vi "start_sweep.vi"(8 "error in (no error)":errorcluster, 11 "ScanModeDL090923Scaffold in":refnum<class "ImagingModeDL090923Scaffold.lvclass">) -> (0 "error out":errorcluster, 3 "ScanModeDL090923Scaffold out":refnum<class "ImagingModeDL090923Scaffold.lvclass">)   [LabVIEW 2010, in "ImagingModeDL090923Scaffold.lvclass"]
uses:
  ImagingModeDL090923Scaffold.lvclass
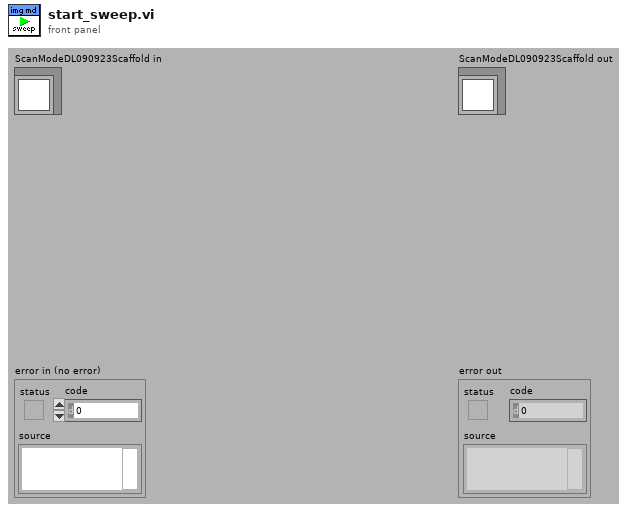
[diagram p1: front panel]
types:
  T1 = typedef "GenericToplevelComponent.lvclass/common_trigger_enum.ctl" = enum16{"NULL", "initialise", "terminate", "fetch command", "fetch data", "attach observer", "register as observer", "detach observer", "acknowledge", "start", "stop", "sweep started", "sweep finished", "experiment started", "experiment stopped"}
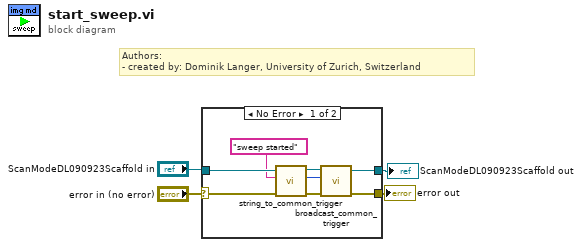
[diagram p0: block diagram]
diagram:
  # "Authors: \n- created by: Dominik Langer, University of Zurich, Switzerland"
  n1 = case shown="No Error" "error in (no error)" {
    selector: "error in (no error)" -> [w10 w14]
    tunnel: [w12 w14] -> w3
    tunnel: [w11 w13] -> w1
    tunnel: "ScanModeDL090923Scaffold in" -> [w8 w13]
    frame No Error {
      n2 = call-dynamic "string_to_common_trigger.vi"("error in (no error)"=w10, "trigger string"="sweep started", "GenericToplevelComponent in"=w8) -> ("error out"=w9:errorcluster, "trigger"=w6:T1, "GenericToplevelComponent out"=w7:refnum<class "ImagingModeDL090923Scaffold.lvclass">)  [unwired: 6 in]
      n3 = call-dynamic "broadcast_common_trigger.vi"("error in (no error)"=w9, "trigger"=w6, "GenericToplevelComponent in"=w7) -> ("error out"=w12:errorcluster, "GenericToplevelComponent out"=w11:refnum<class "ImagingModeDL090923Scaffold.lvclass">)  [unwired: 7 in]
    }
    frame Error {
    }
  }
  "error out" <- w3
  "ScanModeDL090923Scaffold out" <- w1
